vi "rs3 get timestamp domain3.vi"(8 "error in (no error)":errorcluster, 11 "frame in":u64) -> (0 "error out":errorcluster, 1 "error":u64, 2 "Timestamp domain":u16(ring) items=["Hardware clock", "System Time", "Count"], 3 "frame out":u64)   [LabVIEW 2017, in "libRealSense3.lvlib"]
doc: "Provides timestamp"
uses:
  <vilib>/addons/RealSense/libRealSense3.lvlib
  <vilib>/addons/RealSense/realsense2.dll
panel:
  # "RS3 Get Timestamp Domain"
  # "(C) Intel Corp. 2017,  AGJ"
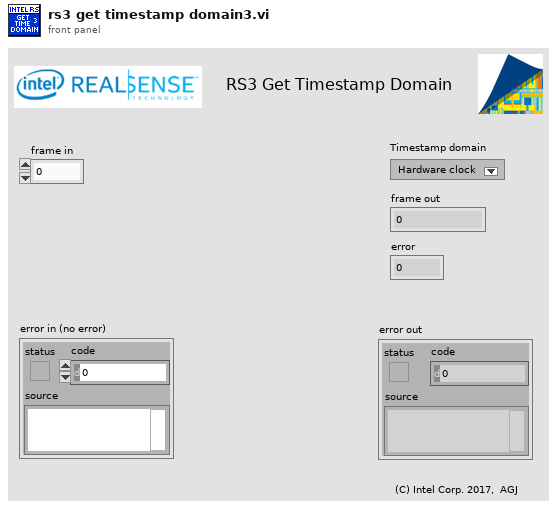
[diagram p1: front panel]
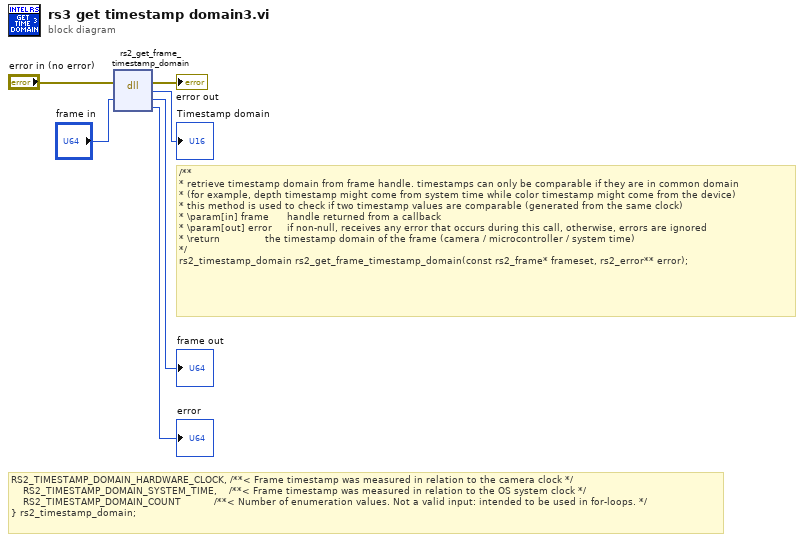
[diagram p0: block diagram]
diagram:
  # "RS2_TIMESTAMP_DOMAIN_HARDWARE_CLOCK, /**< Frame timestamp was measured in relation to the camera clock */\n    RS2_TIMESTAMP_DOMAIN_SYSTEM_TIME,    /**< Frame timestamp was measured in relation to the OS system clock */\n    RS2_TIMESTAMP_DOMAIN_COUNT           /**< Number of enumeration values. Not a valid input: intended to be used in for-loops. */\n} rs2_timestamp_domain;"
  # "/**\n* retrieve timestamp domain from frame handle. timestamps can only be comparable if they are in common domain\n* (for example, depth timestamp might come from system time while color timestamp might come from the device)\n* this method is used to check if two timestamp values are comparable (generated from the same clock)\n* \\param[in] frame      handle returned from a callback\n* \\param[out] error     if non-null, receives any error that occurs during this call, otherwise, errors are ignored\n* \\return               the timestamp domain of the frame (camera / microcontroller / system time)\n*/\nrs2_timestamp_domain rs2_get_frame_timestamp_domain(const rs2_frame* frameset, rs2_error** error);"
  n1 = dll-call lib="C:/Users/agrunnet/Documents/LabVIEW libRealSense5/libRealSense5/realsense2.dll" fn="rs2_get_frame_timestamp_domain"(error in="error in (no error)", "frame"="frame in") -> (error out=→"error out":errorcluster, "timestamp domain"=→"Timestamp domain":u32, "frame"=→"frame out":u64, "error"=→"error":u64)  [unwired: 3 in, 1 out]
